vi "test_libssh2_userauth_keyboard_interactive_ex.vi"() -> ()   [LabVIEW 2017, in "integration_tests.lvlib"]
uses:
  integration_tests.lvlib
  libssh2/libssh2_session_abstract.ctl
  libssh2/libssh2_session_handshake_tcp.vi
  libssh2/libssh2_init_default.vi
  <vilib>/Utility/tcp.llb/TCP Get Raw Net Object.vi
  libssh2/libssh2_session_handshake_socket.vi
  libssh2/libssh2.lvlib
  support/support.lvlib
  <vilib>/PNR/Transparent Assertions/Transparent Assertions/Transparent Assertions.lvlib
panel:
  out "error out":errorcluster
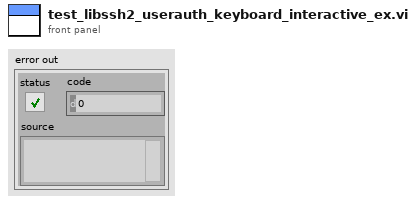
[diagram p1: front panel]
types:
  T1 = typedef "libssh2.lvlib/libssh2_session_abstract.ctl" = cluster{"send":refnum<vi>, "receive":refnum<vi>, "keyboard-interactive response":refnum<vi>}
  T2 = typedef "libssh2.lvlib/Session Refnum.ctl" = refnum<k1>
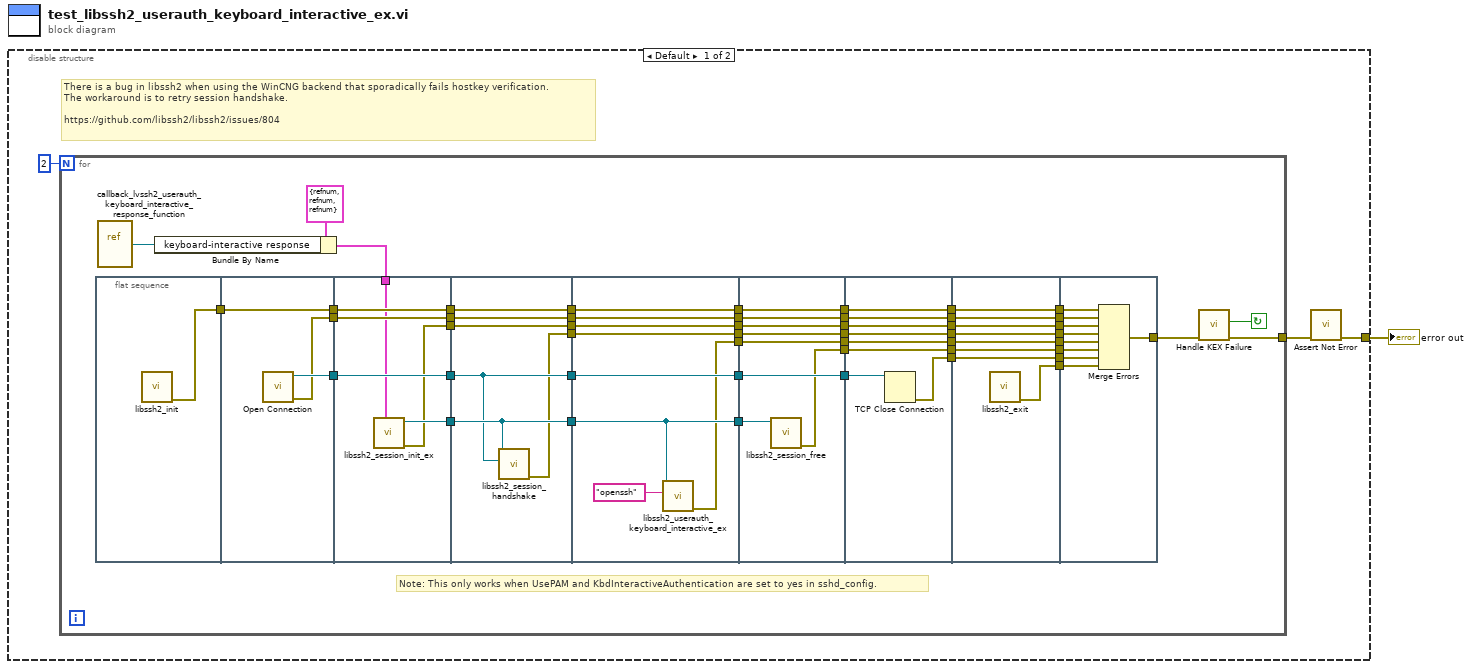
[diagram p0: block diagram]
diagram:
  n1 = disable-structure shown="Default" {
    disable-tunnel: [w4 _] -> w1
    frame condition #0 (active) {
      # "There is a bug in libssh2 when using the WinCNG backend that sporadically fails hostkey verification.\nThe workaround is to retry session handshake.\n\nhttps://github.com/libssh2/libssh2/issues/804"
      n2 = for {
        N: 2 -> [_]
        tunnel: [w9] -> w3
        stop <- w10 continue-if-true
        # "Note: This only works when UsePAM and KbdInteractiveAuthentication are set to yes in sshd_config."
        n3 = flat-sequence {
          tunnel: [w55] -> w54
          tunnel: [w58] -> w53
          tunnel: w54 -> [w57]
          tunnel: [w57] -> w52
          tunnel: [w56] -> w51
          tunnel: w53 -> [w64]
          tunnel: [w64] -> w50
          tunnel: w52 -> [w63]
          tunnel: [w63] -> w49
          tunnel: w51 -> [w62]
          tunnel: [w62] -> w48
          tunnel: [w61] -> w47
          tunnel: [w60] -> w46
          tunnel: w13 -> [w59]
          tunnel: w50 -> [w66]
          tunnel: [w66] -> w45
          tunnel: w49 -> [w70]
          tunnel: [w70] -> w44
          tunnel: w48 -> [w69]
          tunnel: [w69] -> w43
          tunnel: [w68] -> w42
          tunnel: w47 -> [w68]
          tunnel: w46 -> [w67]
          tunnel: [w67] -> w41
          tunnel: [w65] -> w40
          tunnel: w45 -> [w78]
          tunnel: [w78] -> w39
          tunnel: w44 -> [w77]
          tunnel: [w77] -> w38
          tunnel: w43 -> [w76]
          tunnel: [w76] -> w37
          tunnel: w42 -> [w73]
          tunnel: w41 -> [w75]
          tunnel: [w75] -> w36
          tunnel: w40 -> [w74]
          tunnel: [w74] -> w35
          tunnel: [w73] -> w34
          tunnel: [w71] -> w8
          tunnel: w39 -> [w86]
          tunnel: [w86] -> w33
          tunnel: w38 -> [w85]
          tunnel: [w85] -> w32
          tunnel: w37 -> [w84]
          tunnel: [w84] -> w31
          tunnel: w36 -> [w83]
          tunnel: [w83] -> w30
          tunnel: w35 -> [w82]
          tunnel: [w82] -> w29
          tunnel: [w81] -> w28
          tunnel: w34 -> [w80]
          tunnel: w8 -> [w79]
          tunnel: [w79] -> w7
          tunnel: w33 -> [w94]
          tunnel: w32 -> [w93]
          tunnel: [w93] -> w27
          tunnel: w31 -> [w92]
          tunnel: [w92] -> w26
          tunnel: [w91] -> w25
          tunnel: w30 -> [w90]
          tunnel: [w90] -> w24
          tunnel: w29 -> [w89]
          tunnel: [w89] -> w23
          tunnel: [w88] -> w22
          tunnel: w28 -> [w88]
          tunnel: w7 -> [w87]
          tunnel: [w87] -> w6
          tunnel: w27 -> [w102]
          tunnel: [w102] -> w21
          tunnel: w26 -> [w101]
          tunnel: [w101] -> w20
          tunnel: w25 -> [w100]
          tunnel: [w100] -> w19
          tunnel: [w99] -> w18
          tunnel: w24 -> [w98]
          tunnel: [w98] -> w17
          tunnel: w23 -> [w97]
          tunnel: [w97] -> w16
          tunnel: [w96] -> w15
          tunnel: w22 -> [w96]
          tunnel: w6 -> [w95]
          tunnel: [w95] -> w5
          tunnel: w21 -> [w111]
          tunnel: w20 -> [w110]
          tunnel: w19 -> [w109]
          tunnel: w18 -> [w108]
          tunnel: w17 -> [w107]
          tunnel: w16 -> [w106]
          tunnel: w15 -> [w105]
          tunnel: [w104] -> w11
          tunnel: w5 -> [w103]
          frame #0 {
            n4 = call-poly "libssh2_init.vi"() -> ("error out"=w55:errorcluster)  [unwired: 11 in]
          }
          frame #1 {
            n5 = call "Open Connection.vi"() -> ("error out"=w56:errorcluster, "connection ID"=w58:refnum<k5>)  [unwired: 10 in]
          }
          frame #2 {
            n6 = call "libssh2_session_init_ex.vi"("abstract"=w59) -> ("error out"=w60:errorcluster, "session"=w61:T2)  [unwired: 9 in]
          }
          frame #3 {
            n7 = call-poly "libssh2_session_handshake.vi"("tcp connection"=w66, "session"=w68) -> ("error out"=w65:errorcluster)  [unwired: 9 in]
          }
          frame #4 {
            n8 = call "libssh2_userauth_keyboard_interactive_ex.vi"("username"="openssh", "session"=w73) -> ("error out"=w71:errorcluster)  [unwired: 9 in]
          }
          frame #5 {
            n9 = call "libssh2_session_free.vi"("session"=w80) -> ("error out"=w81:errorcluster)  [unwired: 10 in]
          }
          frame #6 {
            n10 = TCP Close Connection(connection ID=w94) -> (error out=w91:errorcluster)  [unwired: 2 in, 1 out]
          }
          frame #7 {
            n11 = call "libssh2_exit.vi"() -> ("error out"=w99:errorcluster)  [unwired: 11 in]
          }
          frame #8 {
            n12 = Merge Errors(w111, w110, w107, w106, w103, w105, w109, w108) -> (w104:errorcluster)
          }
        }
        n13 = vi-ref "callback_lvssh2_userauth_keyboard_interactive_response_function.vi"() -> (w12:refnum<vi>)
        n14 = Bundle By Name(cluster=T1 {"send"=refnum, "receive"=refnum, "keyboard-interactive response"=refnum} ("abstract"), "keyboard-interactive response"=w12) -> (w13:T1)
        n15 = call "Handle KEX Failure.vi"("error in (no error)"=w11) -> ("error out"=w9:errorcluster, "KEX Failure"=w10:bool)  [unwired: 9 in]
      }
      n16 = call <vilib>:"Assert Not Error.vi"("error in (no error)"=w3) -> ("error out"=w4:errorcluster)  [unwired: 10 in]
    }
    frame condition #1 {
    }
  }
  "error out" <- w1
